vi "Start Lot Admin.vi"() -> (1 "Load Custom FW":bool, 2 "Customer Credentials Output":bool, 3 "Debug Mode Output":bool, 4 "Ok Output":bool, 5 "Custom FW Filename":string, 7 "Lot ID Output":string)   [LabVIEW 2018]
panel:
  in  "Cancel Button":bool
  in  "Ok Button":bool
  in  "Customer Credentials":bool
  in  "Debug Mode":bool
  in  "Custom FW":path
  in  "Lot ID":string
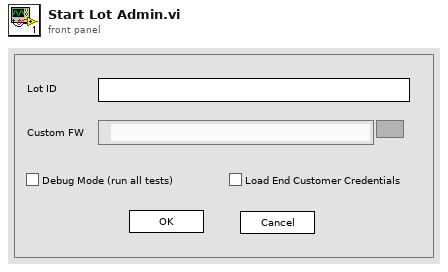
[diagram p1: front panel]
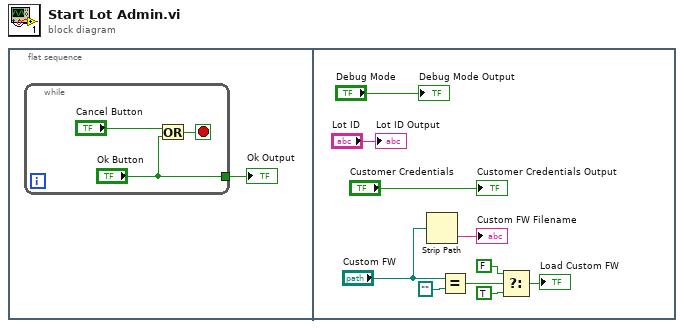
[diagram p0: block diagram]
diagram:
  n1 = flat-sequence {
    frame #0 {
      n2 = while {
        tunnel: ["Ok Button"] -> w1
        stop <- w3 stop-if-true
        n3 = Or(x="Cancel Button", y="Ok Button") -> (x .or. y?=w3:bool)
      }
      "Ok Output" <- w1
    }
    frame #1 {
      n4 = Strip Path(path="Custom FW") -> (name=→"Custom FW Filename":string)  [unwired: 1 out]
      n5 = Equal?(x="Custom FW", y=path "") -> (x = y?=w10:bool)
      n6 = Select(t=FALSE, s=w10, f=TRUE) -> (s? t:f=→"Load Custom FW":bool)
      "Debug Mode Output" <- "Debug Mode"
      "Customer Credentials Output" <- "Customer Credentials"
      "Lot ID Output" <- "Lot ID"
    }
  }
